vi "RIO CAN Frame to Table on PC.vi"(5 "Boolean":bool, 7 "Hexadecimal?":bool, 9 "timestamp":timestamp, 10 "Input Array":string[][](array[string]), 11 "CAN frame":T1 {"type" items=["CAN Data", "CAN Remote"]; "identifier" format="%.0x"}) -> (0 "Numeric":dbl, 2 "string":string, 3 "Output Array":string[][](array[string]), 4 "tekst":string, 6 "okres 100":dbl)   [LabVIEW 2015]
doc: "This example shows how to put a CAN transceiver to sleep on RIO Embedded CAN devices."
uses:
  CANFrameControl.ctl
panel:
  out "string 2":string
  out "substring before match":string
  out "subarray 2":string[](array[string])
  out "subarray":string[](array[string])
  in  "Array":T1[](array[typedef]) {"type" items=["CAN Data", "CAN Remote"]; "identifier" format="%.0x"}
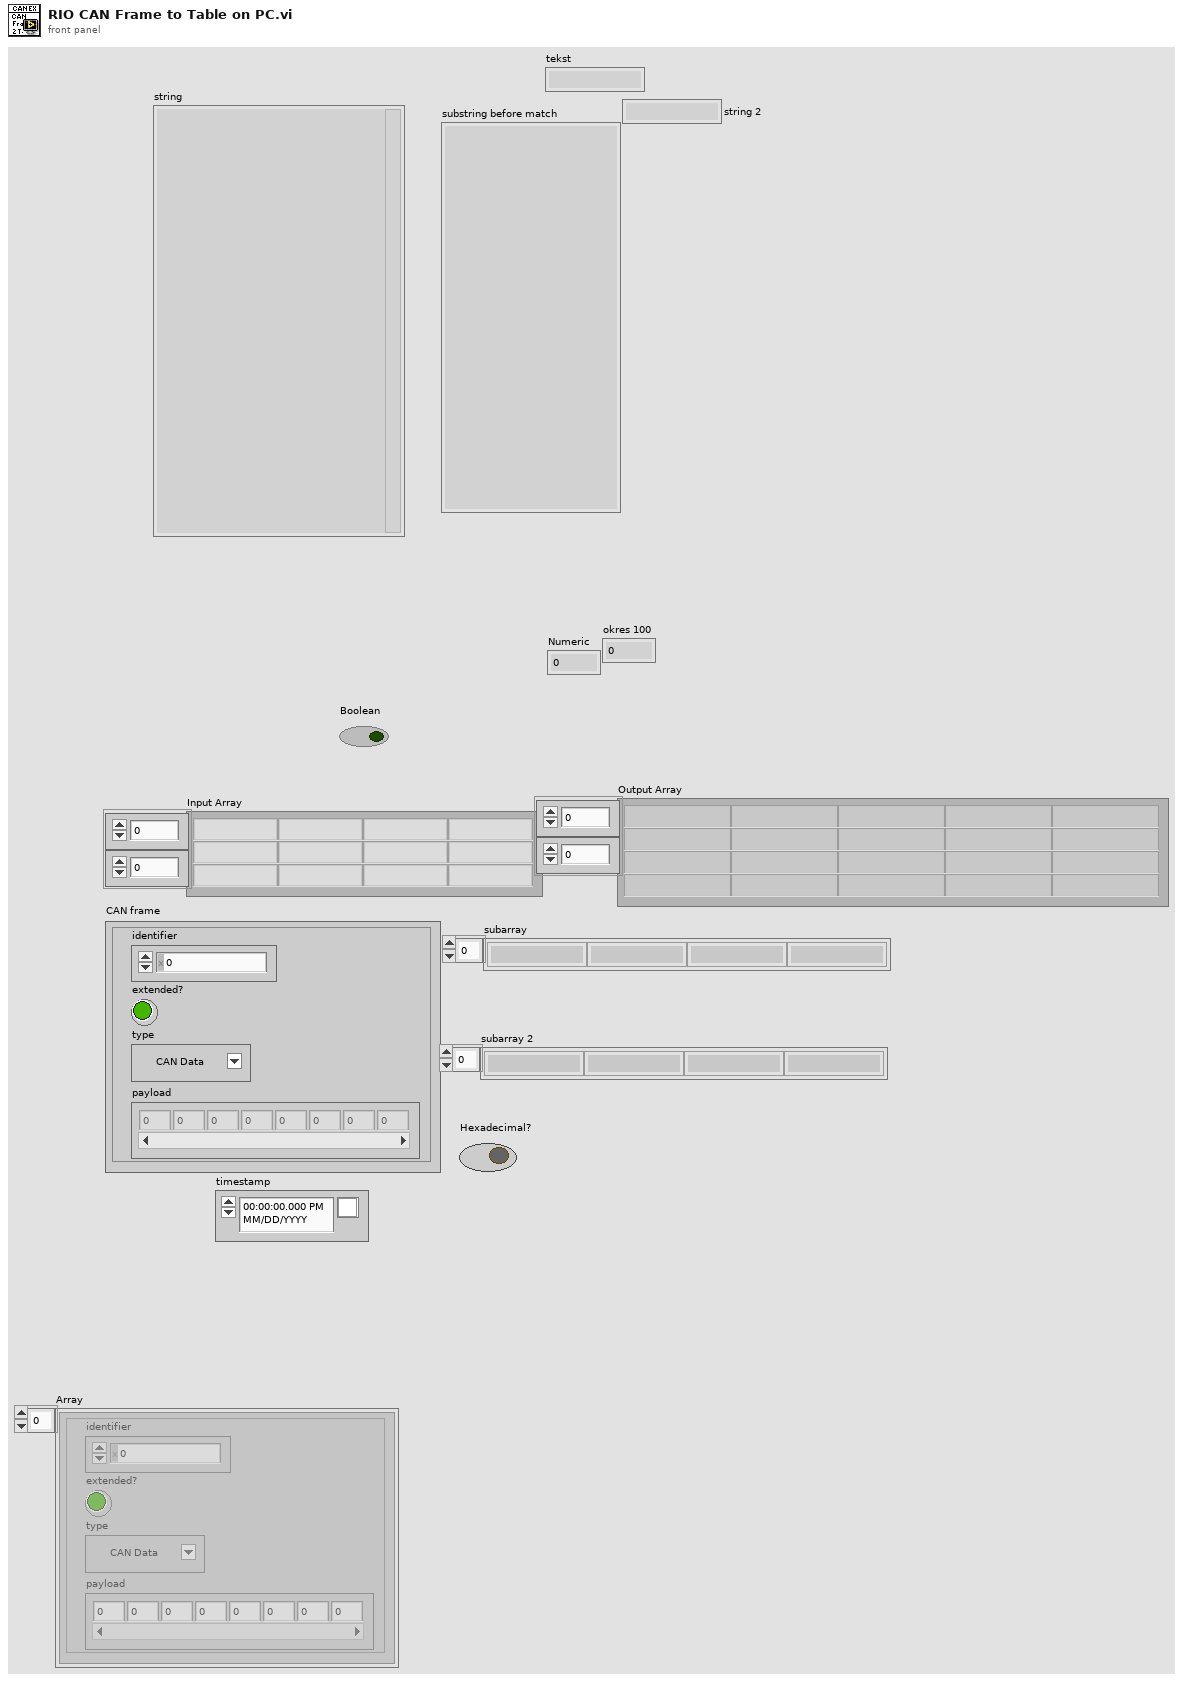
[diagram p1: front panel]
types:
  T1 = typedef "CANFrameControl.ctl" = cluster{"identifier":u32, "extended?":bool, "type":u8, "payload":u8[]}
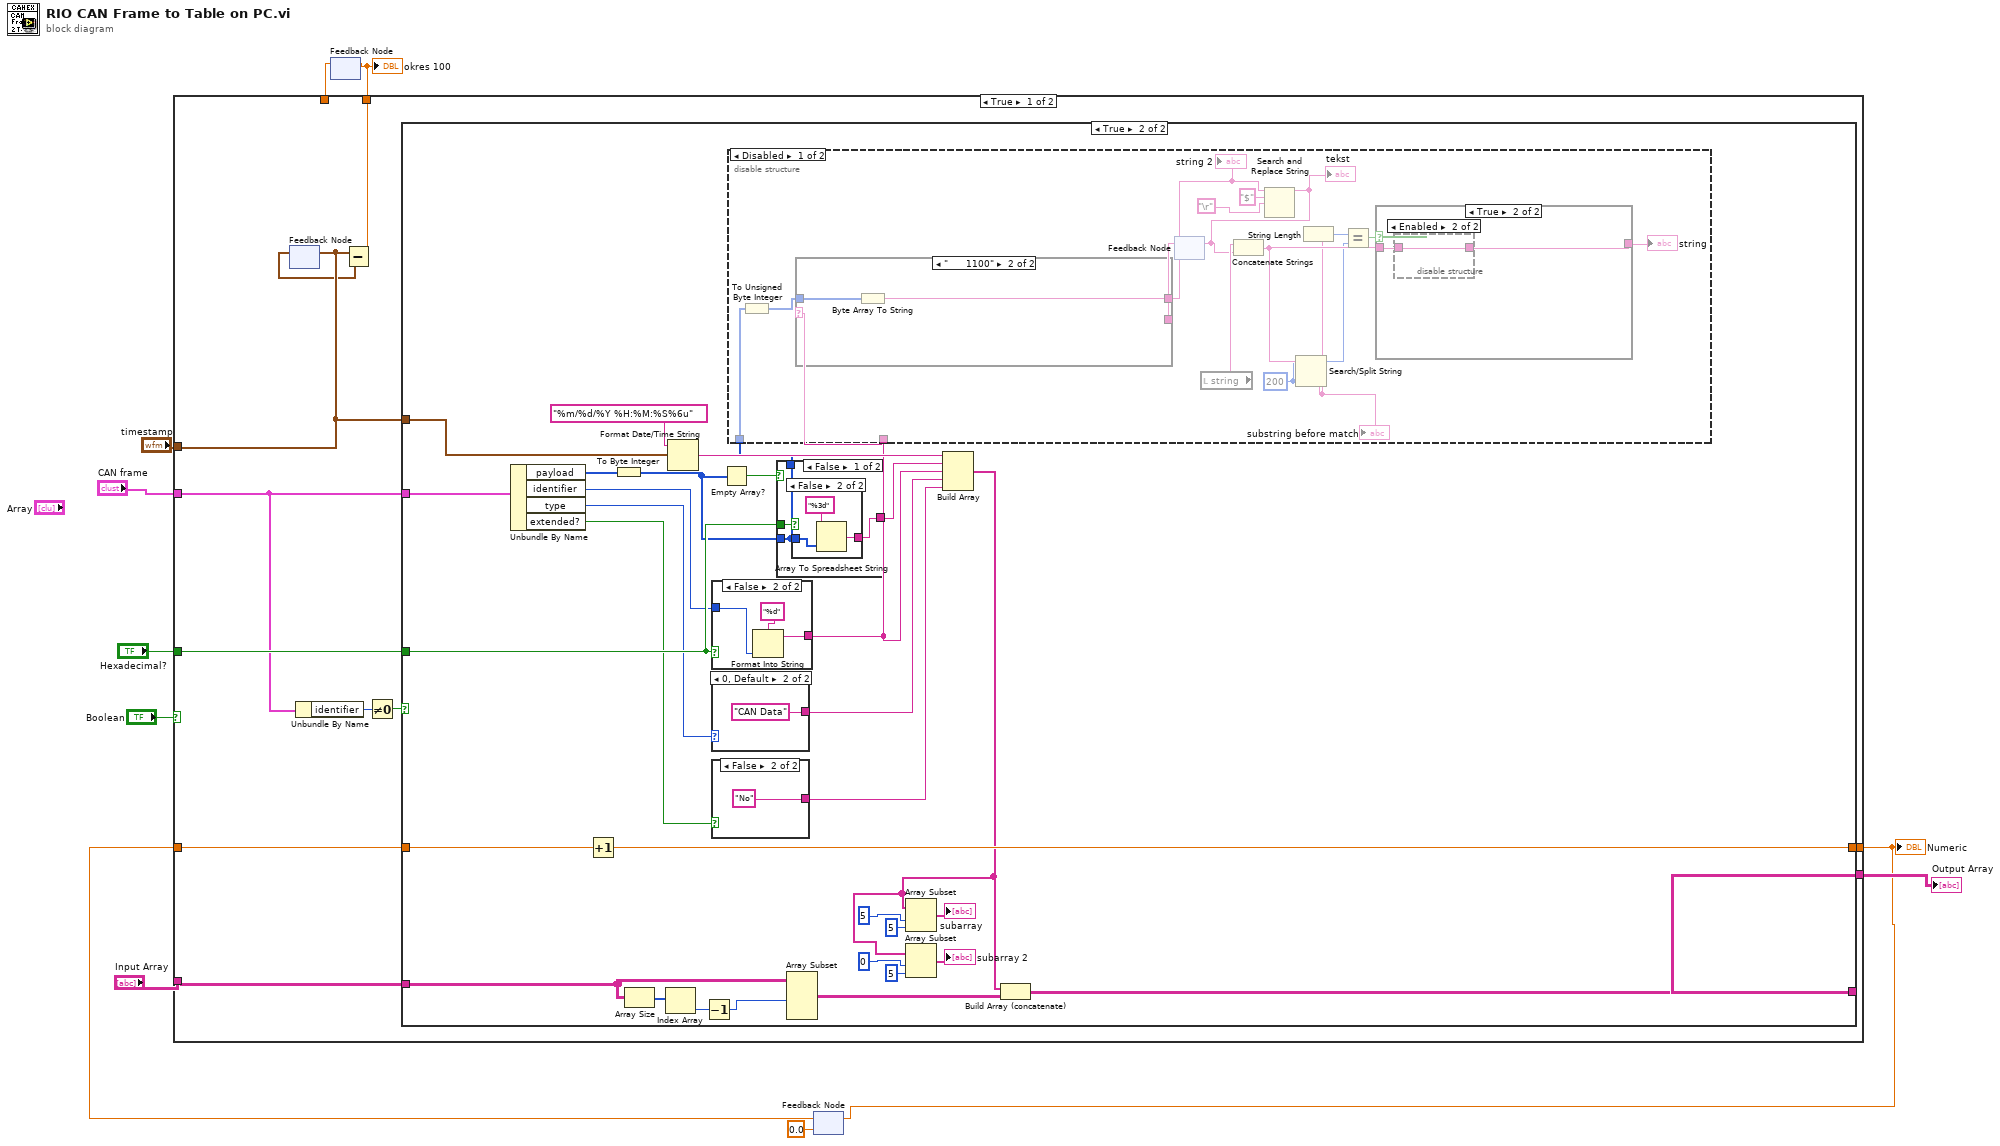
[diagram p0: block diagram]
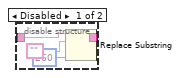
[diagram p4: hidden frame]
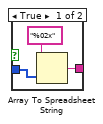
[diagram p7: hidden frame]
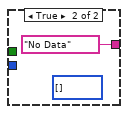
[diagram p8: hidden frame]
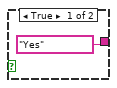
[diagram p9: hidden frame]
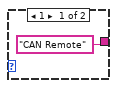
[diagram p10: hidden frame]
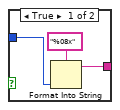
[diagram p11: hidden frame]
diagram:
  n1 = feedback #1() -> (w4:dbl)  [unwired: 1 in]
  n2 = feedback #2(0.0) -> (w3:dbl)
  n3 = case shown="True" "Boolean" {
    tunnel: "Input Array" -> [w20 w104]
    tunnel: [w22 w104] -> w8
    tunnel: "Hexadecimal?" -> [w21 _]
    tunnel: "CAN frame" -> [w17 _]
    tunnel: "timestamp" -> [w14 _]
    tunnel: [w19 w103] -> w2
    tunnel: w3 -> [w18 w103]
    tunnel: [w15 w102] -> w5
    tunnel: w4 -> [_ w102]
    frame True {
      n4 = feedback #3() -> (w13:timestamp)  [unwired: 1 in]
      n5 = feedback-in #3(w14) -> ()
      n6 = Unbundle By Name(w17) -> ("identifier"=w12:u32)
      n7 = Subtract(x=w14, y=w13) -> (x-y=w15:dbl)
      n8 = Not Equal To 0?(x=w12) -> (x != 0?=w16:bool)
      n9 = case shown="True" w16 {
        tunnel: [w23 w55] -> w22
        tunnel: w21 -> [_ w54]
        tunnel: w14 -> [_ w29]
        tunnel: w20 -> [w23 w53]
        tunnel: w17 -> [_ w52]
        tunnel: [w24 w51] -> w19
        tunnel: w18 -> [w24 w50]
        frame False {
        }
        frame True {
          n10 = Unbundle By Name(w52) -> ("payload"=w26:u8[], "identifier"=w30:u32, "type"=w39:u8, "extended?"=w36:bool)
          n11 = Increment(x=w50) -> (x+1=w51:dbl)
          n12 = To Byte Integer(number=w26) -> (8bit integer=w25:i8[])
          n13 = Array Size(array=w53) -> (size(s)=w49:i32[])
          n14 = Index Array(array=w49) -> (element=w48:i32)  [unwired: 1 in]
          n15 = Format Date/Time String(time format string (%c)="%m/%d/%Y %H:%M:%S%6u", seconds (now)=w29) -> (date/time string=w40:string)  [unwired: 1 in]
          n16 = Decrement(x=w48) -> (x-1=w31:i32)
          n17 = case shown="False" w54 {
            tunnel: w30 -> [w97 w100]
            tunnel: [w96 w99] -> w28
            frame True {
              n18 = Format Into String(format string="%08x", w97) -> (resulting string=w96:string)  [unwired: 2 in, 1 out]
            }
            frame False {
              n19 = Format Into String(format string="%d", w100) -> (resulting string=w99:string)  [unwired: 2 in, 1 out]
            }
          }
          n20 = case shown="0, Default" w39 {
            tunnel: ["CAN Remote" "CAN Data"] -> w38
            frame 1 {
            }
            frame 0, Default {
            }
          }
          n21 = case shown="False" w36 {
            tunnel: ["Yes" "No"] -> w37
            frame True {
            }
            frame False {
            }
          }
          n22 = Empty Array?(array=w25) -> (empty?=w33:bool)
          n23 = case shown="False" w33 {
            tunnel: [w83 "No Data"] -> w35
            tunnel: w25 -> [w82 _]
            tunnel: w54 -> [w84 _]
            tunnel: [w82 _] -> w27
            frame False {
              n24 = case shown="False" w84 {
                tunnel: w82 -> [w85 w88]
                tunnel: [w86 w89] -> w83
                frame True {
                  n25 = Array To Spreadsheet String(array=w85, 3:"%02x" ("format string")) -> (spreadsheet string=w86:string)  [unwired: 1 in]
                }
                frame False {
                  n26 = Array To Spreadsheet String(array=w88, 3:"%3d" ("format string")) -> (spreadsheet string=w89:string)  [unwired: 1 in]
                }
              }
            }
            frame True {
              (unwired) u8[] [] ("payload")
            }
          }
          n27 = disable-structure shown="Disabled" {
            disable-tunnel: w28 -> [w70 _]
            disable-tunnel: w27 -> [w56 _]
            frame Disabled {
              w58 = 200 ("offset (0)")
              n28 = To Unsigned Byte Integer(number=w56) -> (unsigned 8bit integer=w57:u8[])
              n29 = feedback #4() -> (w69:string)  [unwired: 1 in]
              n30 = case shown="\"      1100\"" w70 {
                tunnel: w57 -> [_ w81]
                tunnel: [w79 w80] -> w66
                tunnel: w69 -> [w79 _]
                frame "False", Default {
                }
                frame "      1100" {
                  n31 = Byte Array To String(unsigned byte array=w81) -> (string=w80:string)
                }
              }
              "string 2" <- w66
              n32 = local read "string"() -> (w64:string)
              n33 = Search and Replace String(input string=w66, search string="$", replace string="\r") -> (result string=w62:string)  [unwired: 5 in, 3 out]
              "tekst" <- w62
              n34 = feedback-in #4(w62) -> ()
              n35 = Concatenate Strings(w64, w62) -> (w63:string)
              n36 = Search/Split String(string=w63, offset (0)=w58) -> (substring before match=w59:string)  [unwired: 1 in, 2 out]
              "substring before match" <- w59
              n37 = String Length(string=w59) -> (length=w61:i32)
              n38 = Equal?(x=w61, y=w58) -> (x = y?=w60:bool)
              n39 = case shown="True" w60 {
                tunnel: [w71 w73] -> w65
                tunnel: w63 -> [w71 w72]
                frame False {
                }
                frame True {
                  n40 = disable-structure shown="Enabled" {
                    disable-tunnel: [w77 w78] -> w73
                    disable-tunnel: w72 -> [w76 w78]
                    frame Disabled {
                      n41 = Replace Substring(2:260 ("length (len. of substring)"), 4:"", 5:w76) -> (1:w77:string)  [unwired: 1 in, 1 out]
                    }
                    frame Enabled {
                    }
                  }
                }
              }
              "string" <- w65
            }
            frame Enabled {
            }
          }
          n42 = Array Subset(array=w53, length (row)=w31) -> (w41:string[][])  [unwired: 3 in]
          n43 = Build Array(w40, w35, w28, w38, w37) -> (w32:string[])
          n44 = Array Subset(array=w32, index=5 ("length"), length=5) -> (→"subarray":string[])
          n45 = Array Subset(array=w32, index=0 ("length"), length=5) -> (→"subarray 2":string[])
          n46 = Build Array (concatenate)(w32, w41) -> (w55:string[][])
        }
      }
    }
    frame False {
    }
  }
  "Output Array" <- w8
  "Numeric" <- w2
  "okres 100" <- w5
  n47 = feedback-in #1(w5) -> ()
  n48 = feedback-in #2(w2) -> ()
